vi "Read Metrics.vi"(8 "error in (no error)":errorcluster, 11 "Default Collector in":refnum<class "Default Collector.lvclass">) -> (0 "error out":errorcluster, 2 "Metrics":map{string, refnum<data-value>}(c390), 3 "Default Collector out":refnum<class "Default Collector.lvclass">)   [LabVIEW 2020, in "Collector.lvlib" / "Default Collector.lvclass"]
uses:
  Default Collector.lvclass
  metrics/metric/Metric.lvclass
  Default Collector.lvclass/Default Collector.ctl
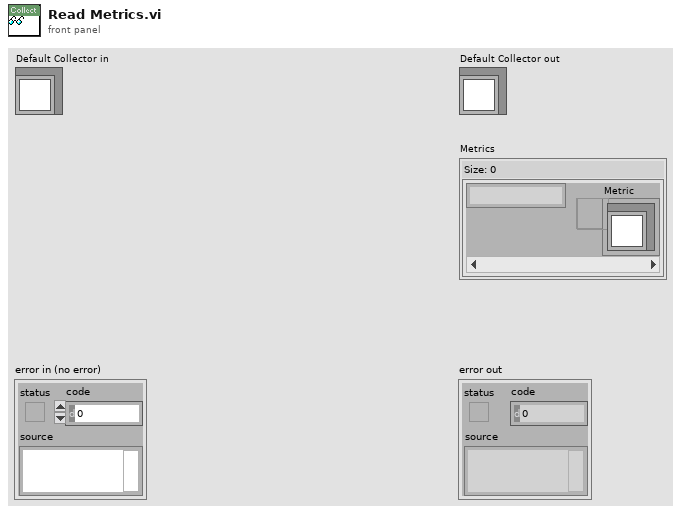
[diagram p1: front panel]
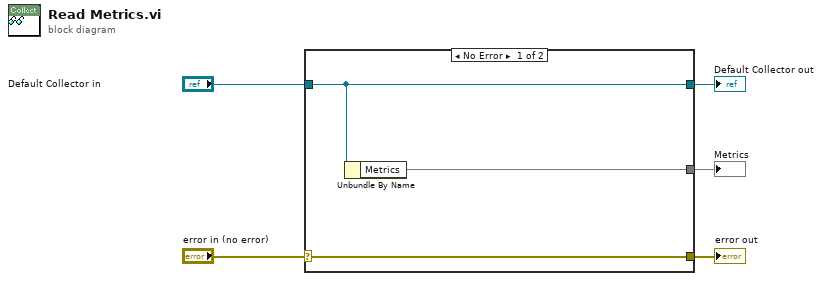
[diagram p0: block diagram]
diagram:
  n1 = case shown="No Error" "error in (no error)" {
    selector: "error in (no error)" -> [w8 w9]
    tunnel: [w8 w9] -> w4
    tunnel: [w7 w10] -> w2
    tunnel: "Default Collector in" -> [w7 w10]
    tunnel: [w6 _] -> w1
    frame No Error {
      n2 = Unbundle By Name(w7) -> ("Metrics"=w6:map{string, refnum<data-value>})
    }
    frame Error {
    }
  }
  "error out" <- w4
  "Default Collector out" <- w2
  "Metrics" <- w1
